vi "Scripting_LibraryInfoMemory.vi"(8 "error in (no error)":errorcluster, 10 "ViPath":path, 11 "Action":T2(ring)) -> (0 "error out":errorcluster, 1 "Found":bool, 2 "LibraryQualifiedName":string, 3 "LibraryName":string, 5 "LibaryPath":path)   [LabVIEW 2012]
panel:
  out "Array":T1(array[cluster])
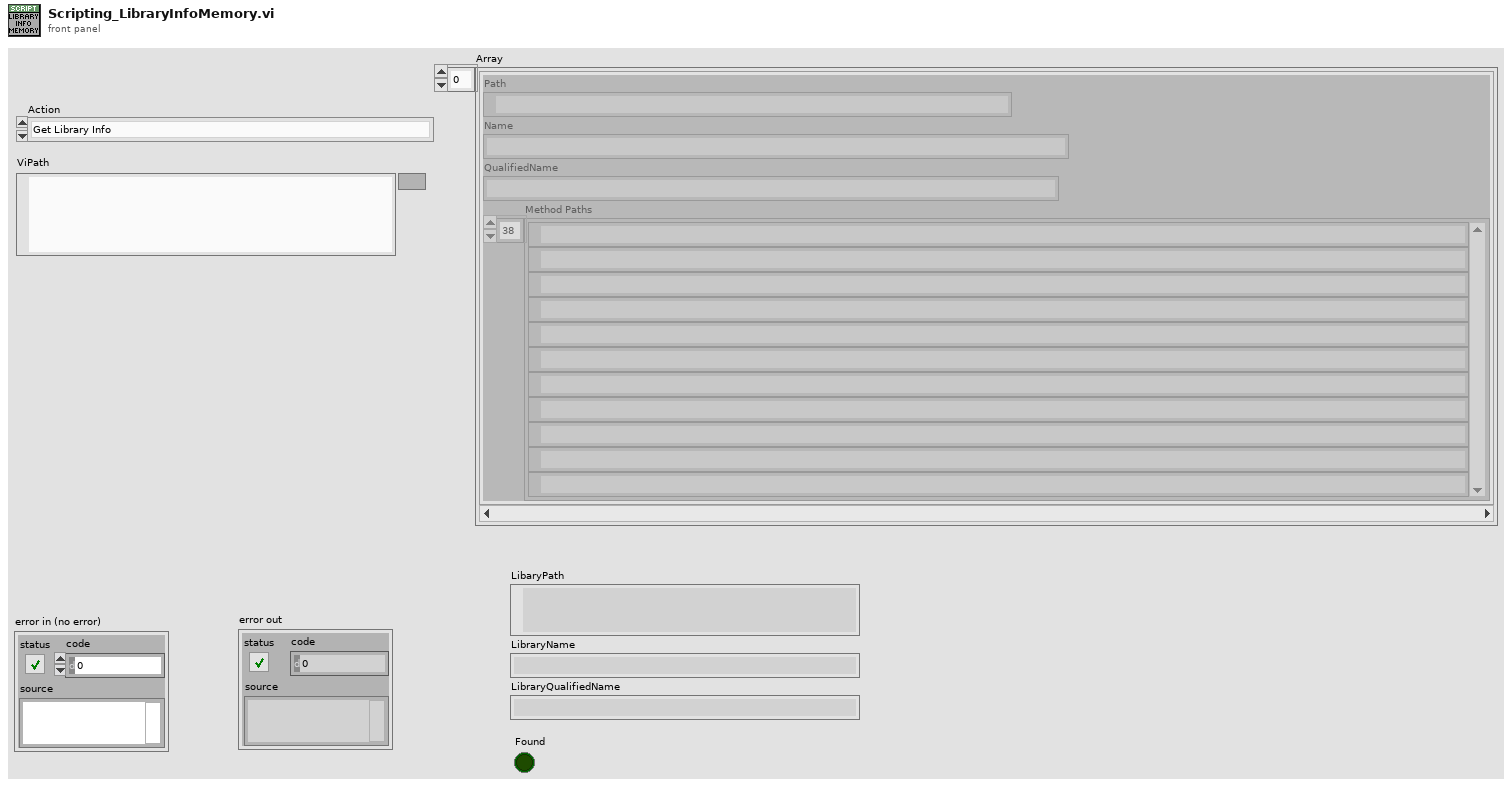
[diagram p1: front panel]
types:
  T1 = cluster{"Path":path, "Name":string, "QualifiedName":string, "Method Paths":path[]}[]
  T2 = enum16{"Get Library Info", "Create Library Info", "Clear Library Info"}
  T3 = cluster{"Path":path, "Name":string, "QualifiedName":string, "Methods":path[]}[]
  T4 = enum32{"invalid scope", "public", "private", "protected", "community"}
  T5 = enum32{"invalid scope", "public", "private", "protected", "community"}[]
  T6 = cluster{"Path":path, "Name":string, "QualifiedName":string, path[]}
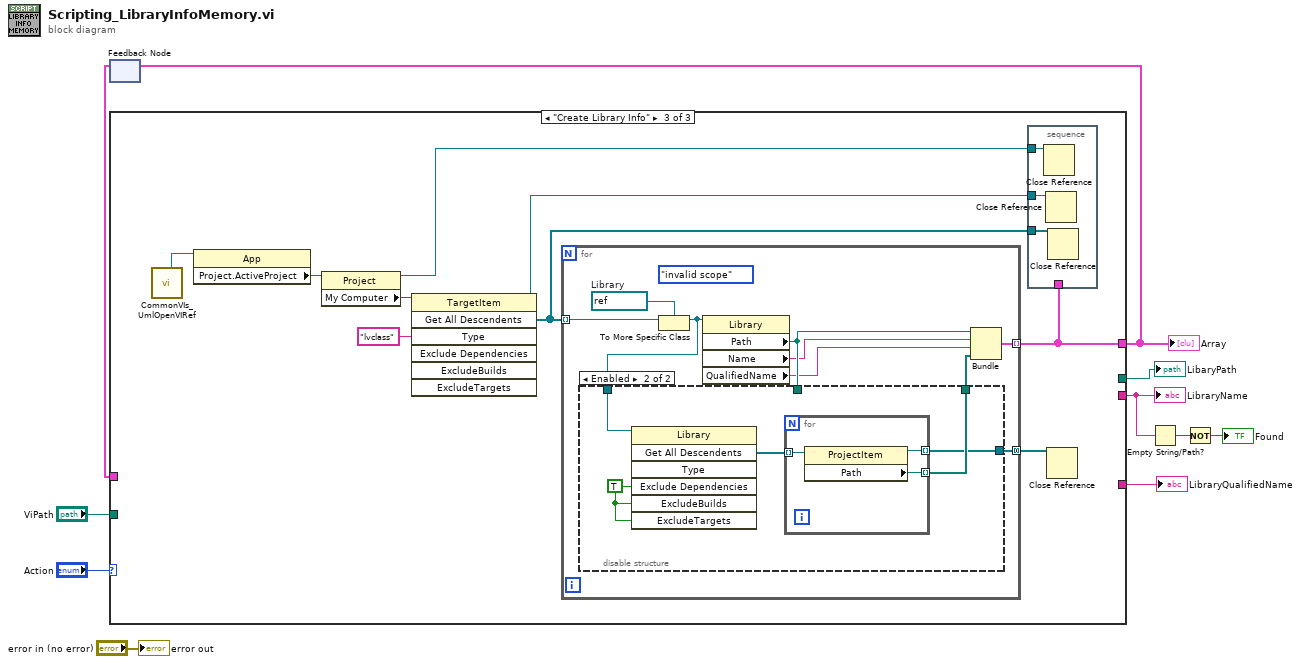
[diagram p0: block diagram]
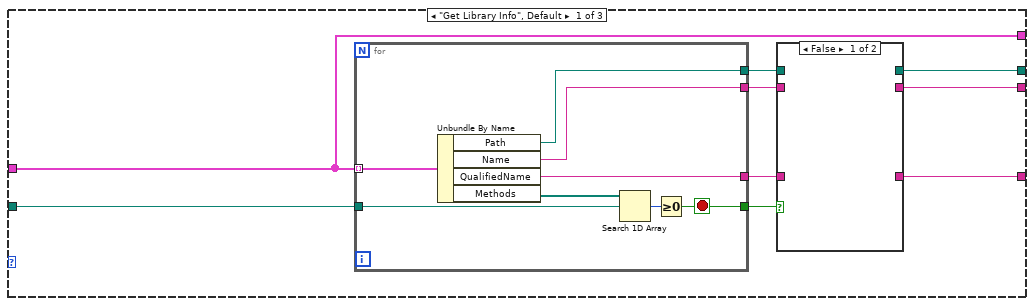
[diagram p2: hidden frame]
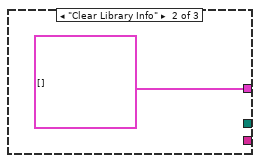
[diagram p4: hidden frame]
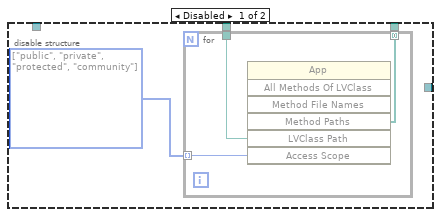
[diagram p5: hidden frame]
diagram:
  n1 = feedback #1() -> (w8:T3)  [unwired: 1 in]
  n2 = case shown="\"Create Library Info\"" "Action" {
    tunnel: [w19 T3 [] w34] -> w4
    tunnel: w8 -> [w19 _ _]
    tunnel: "ViPath" -> [w18 _ _]
    tunnel: [w13 _ _] -> w6
    tunnel: [w12 _ _] -> w3
    tunnel: [w11 _ _] -> w5
    frame "Get Library Info", Default {
      n3 = for {
        tunnel: w19 -> [w30] mode=indexing
        tunnel: w18 -> [w29]
        tunnel: [w27] -> w16
        tunnel: [w26] -> w15
        tunnel: [w25] -> w14
        tunnel: [w24] -> w17
        stop <- w24 stop-if-true
        n4 = Unbundle By Name(w30) -> ("Path"=w27:path, "Name"=w26:string, "QualifiedName"=w25:string, "Methods"=w23:path[])
        n5 = Search 1D Array(1D array=w23, element=w29) -> (index of element=w28:i32)  [unwired: 1 in]
        n6 = Greater Or Equal To 0?(x=w28) -> (x >= 0?=w24:bool)
      }
      n7 = case shown="False" w17 {
        tunnel: w16 -> [_ w22]
        tunnel: w15 -> [_ w21]
        tunnel: w14 -> [_ w20]
        tunnel: [_ w22] -> w13
        tunnel: [_ w21] -> w12
        tunnel: [_ w20] -> w11
        frame False {
        }
        frame True {
        }
      }
    }
    frame "Clear Library Info" {
    }
    frame "Create Library Info" {
      n8 = call <resource>:"CommonVIs_UmlOpenVIRef.vi"() -> ("AppRefOut"=w40:refnum<vi>)  [unwired: 8 in, 3 out]
      n9 = property class="App"(reference=w40) -> ("Project.ActiveProject"=w39:refnum<vi>)  [unwired: 1 in, 2 out]
      n10 = property class="Project"(reference=w39) -> (reference out=w32:refnum<vi>, "My Computer"=w37:refnum<vi>)  [unwired: 1 in, 1 out]
      n11 = invoke class="TargetItem" method="Get All Descendents"(reference=w37, "Type"="lvclass") -> (reference out=w33:refnum<vi>, "All Descendents"=w35:refnum<vi>[])  [unwired: 5 in, 5 out]
      n12 = for {
        tunnel: w35 -> [w52] mode=indexing
        tunnel: [w46] -> w34 mode=indexing
        tunnel: [w44] -> w36 mode=concatenating
        w51 = refnum<vi> refnum  # Library
        (unwired) T4."invalid scope" ("Access Scope")
        n13 = To More Specific Class(target class=w51, reference=w52) -> (specific class reference=w45:refnum<vi>)  [unwired: 1 in, 1 out]
        n14 = property class="Library"(reference=w45) -> ("Path"=w50:path, "Name"=w49:string, "QualifiedName"=w48:string)  [unwired: 1 in, 2 out]
        n15 = disable-structure shown="Enabled" {
          disable-tunnel: w50 -> [w55 _]
          disable-tunnel: [w54 w61] -> w47
          disable-tunnel: w45 -> [_ w63]
          disable-tunnel: [_ w60] -> w44
          frame Disabled {
            w53 = T5 [enum."public", enum."private", enum."protected", enum."community"] items=["invalid scope", "public", "private", "protected", "community"]
            n16 = for {
              tunnel: w55 -> [w58]
              tunnel: [w57] -> w54 mode=concatenating
              tunnel: w53 -> [w56] mode=indexing
              n17 = invoke class="App" method="All Methods Of LVClass"("LVClass Path"=w58, "Access Scope"=w56) -> ("Method Paths"=w57:path[])  [unwired: 5 in, 6 out]
            }
          }
          frame Enabled {
            w59 = TRUE ("ExcludeDependencies")
            n18 = invoke class="Library" method="Get All Descendents"(reference=w63, "Exclude Dependencies"=w59, "ExcludeBuilds"=w59, "ExcludeTargets"=w59) -> ("All Descendents"=w62:refnum<vi>[])  [unwired: 3 in, 6 out]
            n19 = for {
              tunnel: w62 -> [w66] mode=indexing
              tunnel: [w65] -> w61 mode=indexing
              tunnel: [w64] -> w60 mode=indexing
              n20 = property class="ProjectItem"(reference=w66) -> (reference out=w64:refnum<vi>, "Path"=w65:path)  [unwired: 1 in, 1 out]
            }
          }
        }
        n21 = Bundle("Path"=w50, "Name"=w49, "QualifiedName"=w48, w47) -> (w46:T6)  [unwired: 1 in]
      }
      n22 = stacked-sequence {
        tunnel: w35 -> [w43]
        tunnel: w34 -> [_]
        tunnel: w33 -> [w42]
        tunnel: w32 -> [w41]
        frame #0 {
          n23 = Close Reference(reference=w41) -> ()  [unwired: 1 in, 1 out]
          n24 = Close Reference(reference=w42) -> ()  [unwired: 1 in, 1 out]
          n25 = Close Reference(reference=w43) -> ()  [unwired: 1 in, 1 out]
        }
      }
      n26 = Close Reference(reference=w36) -> ()  [unwired: 1 in, 1 out]
    }
  }
  "LibraryQualifiedName" <- w5
  "LibraryName" <- w3
  "LibaryPath" <- w6
  "Array" <- w4
  n27 = feedback-in #1(w4) -> ()
  n28 = Empty String/Path?(string/path=w3) -> (empty?=w2:bool)
  n29 = Not(x=w2) -> (.not. x?=→"Found":bool)
  "error out" <- "error in (no error)"
